vi "C4Dev_unregisterEvent.vi"(0 "c4dev in":refnum<k24>, 5 "name in":string, 11 "error in":errorcluster) -> (4 "c4dev out":refnum<k24>, 15 "error out":errorcluster)   [LabVIEW 2015, in "libC4HdlLV.lvlib"]
uses:
  libC4HdlLV.lvlib
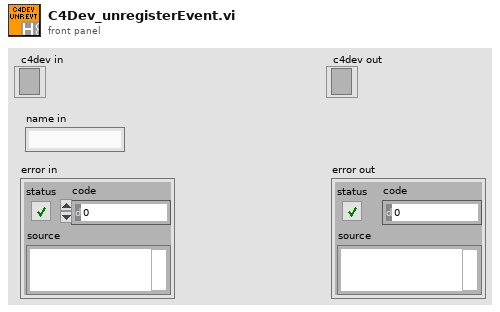
[diagram p1: front panel]
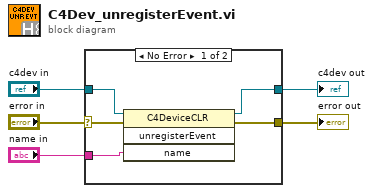
[diagram p0: block diagram]
diagram:
  n1 = case shown="No Error" "error in" {
    selector: "error in" -> [w8 w12]
    tunnel: [w7 w12] -> w4
    tunnel: "c4dev in" -> [w10 w11]
    tunnel: [w9 w11] -> w2
    tunnel: "name in" -> [w6 _]
    frame No Error {
      n2 = invoke class="C4DeviceCLR" method="unregisterEvent"(reference=w10, error in=w8, "name"=w6) -> (reference out=w9:refnum<k24>, error out=w7:errorcluster)  [unwired: 1 in, 2 out]
    }
    frame Error {
    }
  }
  "error out" <- w4
  "c4dev out" <- w2
